vi "New Test.vi"(8 "error in (no error)":errorcluster) -> (0 "error out":errorcluster)   [LabVIEW 2020, in "MacroAssert.lvlib"]
doc: "Presents an interface to create, edit, save, and execute user-defined macros."
uses:
  MacroAssert.lvlib
  <vilib>/Utility/miscctls.llb/LVRowAndColumnUnsignedTypeDef.ctl
  bd503c13-d10c-440e-ab5e-4e60baef5deb.vi
  SubVIs/FaKI State Machine/FaKI State Machine.lvlib
  CTLs/State Data.ctl
  CTLs/Hotkey Values.ctl
  CTLs/FGV Actions.ctl
  CTLs/Hotkey Type.ctl
  CTLs/Refs.ctl
  CTLs/Step Type V3.ctl
  CTLs/Step V3.ctl
  CTLs/Macro Cluster V3.ctl
  CTLs/Macro Config V3.ctl
  fa5aba67-e91f-4216-ac5c-c17457851557.vi
  CTLs/Assertion Type.ctl
  CTLs/Report Data.ctl
  <vilib>/Utility/inputDevices.llb/closeKeyboard.vi
panel:
  in  "String":string="C:\\Users\\User\\Desktop\\test.txt"
  in  "File Path":path
  out "Status":string
  in  "Add Step 2":bool
  in  "Dbl Click":T1
  in  "Macro Steps":i32(listbox)
  out "Abort Hotkey":string caption="Abort Hotkey:"
  out "Metadata":string
  in  "Description":string
  out "Resolutions":cluster{"Width":i16, "Height":i16}[](array[cluster])
  out "n Monitors":i32
  in  "Settings":bool
  in  "Export":bool
  in  "Import":bool
  out "Macro Hotkey":string caption="Macro Hotkey:"
  in  "Delete":bool
  in  "Start/Stop":bool
  in  "N":i32 caption="Times to Repeat\n(-1 = indefinitely)" min=-1
  in  "Activation Type":enum32{"Hotkey", "Automatic"}(radio)
  out "Row":i32
  in  "Clear Steps":bool
  in  "Delete Step":bool
  in  "Insert Step":bool
  in  "Add Step":bool
  in  "Modify Step":bool
  in  "Exit":bool
  in  "Save":bool
  in  "Restore":bool
  in  "Help":bool
  in  "Macro Name":string(combo)
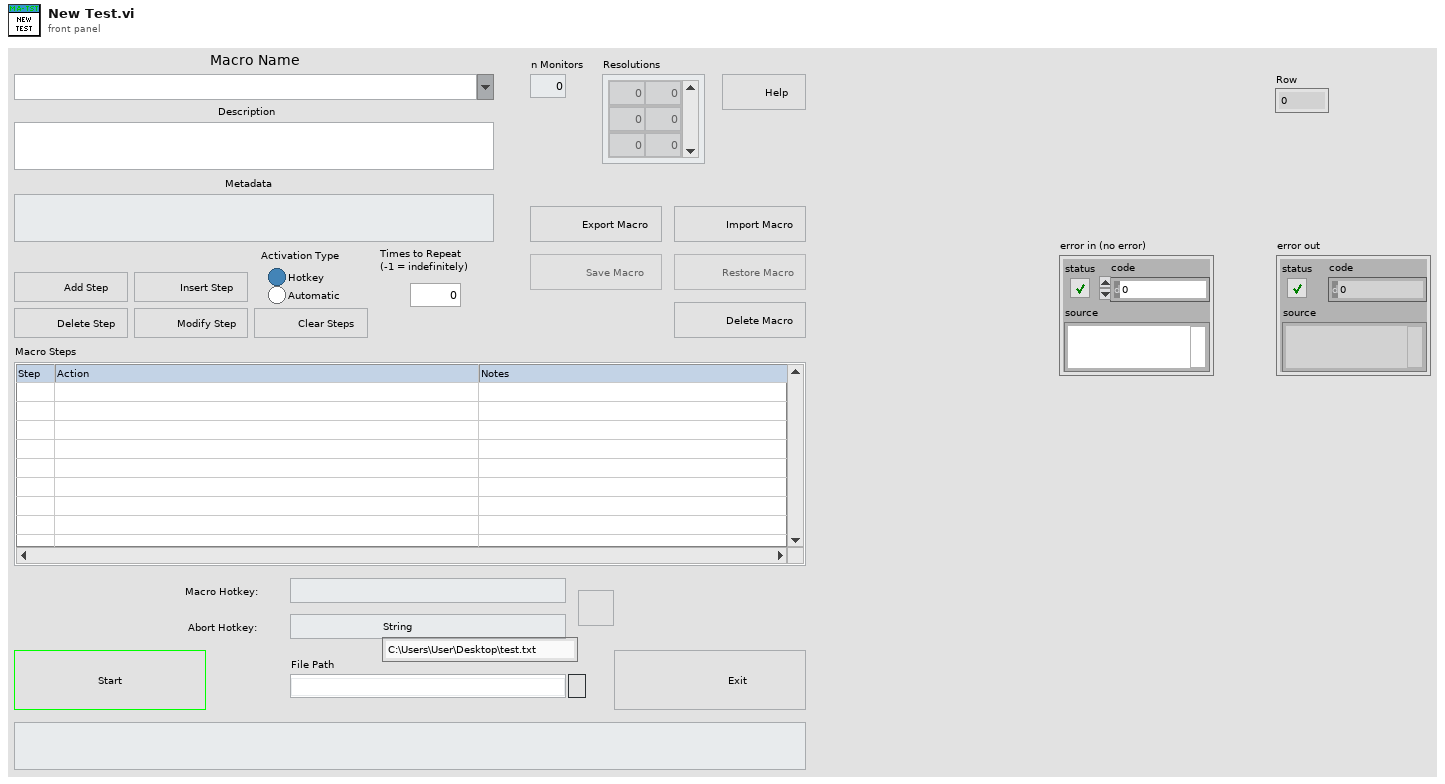
[diagram p1: front panel]
types:
  T1 = cluster{"Insert Before":bool, "Insert After":bool, "Modify Step 2":bool, "Delete Step 2":bool}
  T2 = typedef "LVPoint32TypeDef.ctl" = cluster{"Horizontal":i32, "Vertical":i32}
  T3 = enum32{"Invalid", "Standard", "Closed", "Hidden", "Minimized", "Maximized"}
  T4 = enum32{"invalid app kind", "Development System", "Run Time System", "Student Edition", "Embedded LabVIEW", "Evaluation", "Custom"}
  T5 = typedef "MacroAssert.lvlib/State Data.ctl" = cluster{"Core":cluster{"Current VI Reference":refnum<vi>, "Close Panel on Exit?":bool}, "Macro":cluster{"New":T6, "Saved":T6, "Name":string}, "Step":i32, "n":i32, "Hotkey Values":T11, "Keyboard":refnum<k1>, "Macro Active?":bool, "Macro Names":string[], "Rcount":i32, "Refs":T12, "Resolutions":cluster{"Width":i16, "Height":i16}[], "App Data Dir":path, "Start Time":timestamp, "Report Data":T13[]}
  T6 = typedef "MacroAssert.lvlib/Macro Cluster V3.ctl" = cluster{"Config":T7, "Steps":T8[]}
  T7 = typedef "MacroAssert.lvlib/Macro Config V3.ctl" = cluster{"Schema Version":string, "Activation Type":enum32{"Hotkey", "Automatic"}, "N":i32, "Description":string, "Resolutions":cluster{"Width":i16, "Height":i16}[], "Date Created":timestamp, "Date Updated":timestamp}
  T8 = typedef "MacroAssert.lvlib/Step V3.ctl" = cluster{"Type":T9, "X":i32, "Y":i32, "Delay":i32, "Key":u8, "Repeat":i32, "RClick?":bool, "App/Window Name":string, "Notes":string, "Assertion Type":T10, "Assertion Parameters":variant}
  T9 = typedef "MacroAssert.lvlib/Step Type V3.ctl" = enum16{"Mouse Move", "Mouse Click", "Key Press", "Wait", "Mouse Down", "Mouse Up", "Key Down", "Key Up", "Test Assertion", "Run Application", "Maximize Window", "Restore Window", "Minimize Window", "Close Window", "Bring Window to Front", "Send Window to Back"}
  T10 = typedef "MacroAssert.lvlib/Assertion Type.ctl" = enum16{"Control Position", "Control Visible", "Control Disabled", "Control Image"}
  T11 = typedef "MacroAssert.lvlib/Hotkey Values.ctl" = cluster{"Macro Hotkey":enum16{"0", "1", "2", "3", "4", "5", "6", "7", "8", "9", "A", "B", "C", "D", "E", "F", "G", "H", "I", "J", "K", "L", "M", "N", "O", "P", "Q", "R", "S", "T", "U", "V", "W", "X", "Y", "Z", "F1", "F2", "F3", "F4", "F5", "F6", "F7", "F8", "F9", "F10", "F11", "F12", "F13", "F14", "F15", "ADD", "BACK", "BACKSLASH", "CAPITAL", "COMMA", "DECIMAL", "DELETE", "DIVIDE", "DOWN", "END", "EQUALS", "ESCAPE", "GRAVE (`)", "HOME", "INSERT", "LBRACKET", "LCONTROL", "LEFT", "L ALT", "LSHIFT", "LWIN", "MINUS", "MULTIPLY", "NEXT", "NUMLOCK", "NUMPAD_0", "NUMPAD_1", "NUMPAD_2", "NUMPAD_3", "NUMPAD_4", "NUMPAD_5", "NUMPAD_6", "NUMPAD_7", "NUMPAD_8", "NUMPAD_9", "PAUSE", "PERIOD", "PRIOR (PG UP)", "RBRACKET", "RCONTROL", "RETURN", "RIGHT", "R ALT", "RSHIFT", "RWIN", "SCROLL", "SEMICOLON", "SLASH", "SPACE", "SUBTRACT", "TAB", "UP", "ENTER (num pad)", "' (quote)"}[], "Abort Hotkey":enum16{"0", "1", "2", "3", "4", "5", "6", "7", "8", "9", "A", "B", "C", "D", "E", "F", "G", "H", "I", "J", "K", "L", "M", "N", "O", "P", "Q", "R", "S", "T", "U", "V", "W", "X", "Y", "Z", "F1", "F2", "F3", "F4", "F5", "F6", "F7", "F8", "F9", "F10", "F11", "F12", "F13", "F14", "F15", "ADD", "BACK", "BACKSLASH", "CAPITAL", "COMMA", "DECIMAL", "DELETE", "DIVIDE", "DOWN", "END", "EQUALS", "ESCAPE", "GRAVE (`)", "HOME", "INSERT", "LBRACKET", "LCONTROL", "LEFT", "L ALT", "LSHIFT", "LWIN", "MINUS", "MULTIPLY", "NEXT", "NUMLOCK", "NUMPAD_0", "NUMPAD_1", "NUMPAD_2", "NUMPAD_3", "NUMPAD_4", "NUMPAD_5", "NUMPAD_6", "NUMPAD_7", "NUMPAD_8", "NUMPAD_9", "PAUSE", "PERIOD", "PRIOR (PG UP)", "RBRACKET", "RCONTROL", "RETURN", "RIGHT", "R ALT", "RSHIFT", "RWIN", "SCROLL", "SEMICOLON", "SLASH", "SPACE", "SUBTRACT", "TAB", "UP", "ENTER (num pad)", "' (quote)"}[]}
  T12 = typedef "MacroAssert.lvlib/Refs.ctl" = cluster{"Name":refnum<vi>, "Description":refnum<vi>, "Import":refnum<vi>, "Export":refnum<vi>, "Delete":refnum<vi>, "Restore":refnum<vi>, "Save":refnum<vi>, "Start":refnum<vi>, "Steps":refnum<vi>, "Simple Refs":refnum<vi>[]}
  T13 = typedef "MacroAssert.lvlib/Report Data.ctl" = cluster{"Step":string, "Pass?":bool, "Actual Value":variant}
  T14 = enum8{"Enabled", "Disabled", "Disabled and Grayed Out"}
  T15 = typedef "LVRowAndColumnUnsignedTypeDef.ctl" = cluster{"Row":u32, "Column":u32}
  T16 = typedef "MacroAssert.lvlib/Hotkey Type.ctl" = enum16{"Macro Hotkey", "Abort Hotkey"}
  T17 = typedef "MacroAssert.lvlib/FGV Actions.ctl" = enum16{"Read", "Write"}
  T18 = cluster{"Current VI Reference":refnum<vi>, "Close Panel on Exit?":bool}
  T19 = enum16{"0", "1", "2", "3", "4", "5", "6", "7", "8", "9", "A", "B", "C", "D", "E", "F", "G", "H", "I", "J", "K", "L", "M", "N", "O", "P", "Q", "R", "S", "T", "U", "V", "W", "X", "Y", "Z", "F1", "F2", "F3", "F4", "F5", "F6", "F7", "F8", "F9", "F10", "F11", "F12", "F13", "F14", "F15", "ADD", "BACK", "BACKSLASH", "CAPITAL", "COMMA", "DECIMAL", "DELETE", "DIVIDE", "DOWN", "END", "EQUALS", "ESCAPE", "GRAVE (`)", "HOME", "INSERT", "LBRACKET", "LCONTROL", "LEFT", "L ALT", "LSHIFT", "LWIN", "MINUS", "MULTIPLY", "NEXT", "NUMLOCK", "NUMPAD_0", "NUMPAD_1", "NUMPAD_2", "NUMPAD_3", "NUMPAD_4", "NUMPAD_5", "NUMPAD_6", "NUMPAD_7", "NUMPAD_8", "NUMPAD_9", "PAUSE", "PERIOD", "PRIOR (PG UP)", "RBRACKET", "RCONTROL", "RETURN", "RIGHT", "R ALT", "RSHIFT", "RWIN", "SCROLL", "SEMICOLON", "SLASH", "SPACE", "SUBTRACT", "TAB", "UP", "ENTER (num pad)", "' (quote)"}[]
  T20 = typedef "LVAllMonitorsDisplayTypeDef.ctl" = cluster{"Bounds":cluster{"Left":i16, "Top":i16, "Right":i16, "Bottom":i16}, "Depth":i16}[]
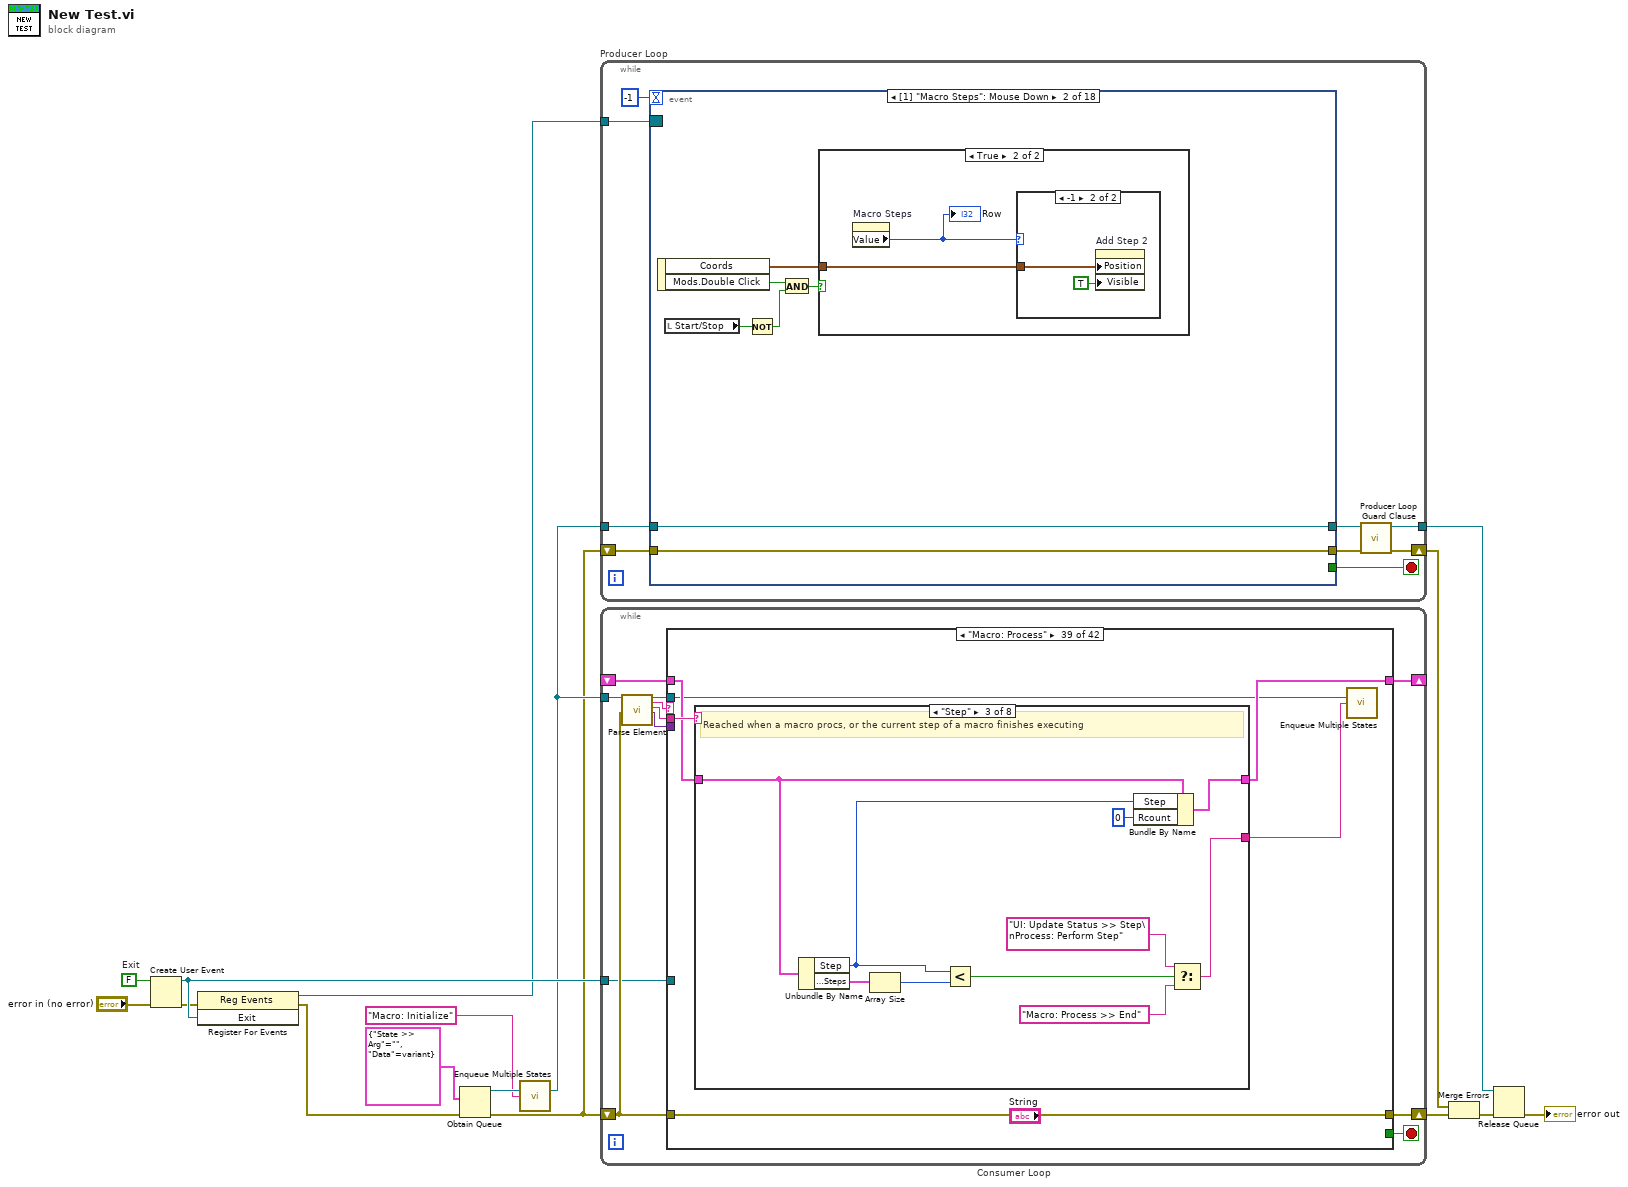
[diagram p0: block diagram]
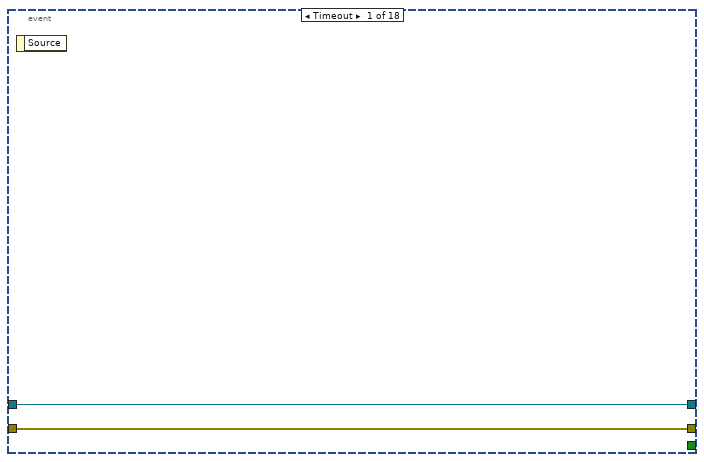
[diagram p2: hidden frame]
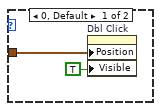
[diagram p4: hidden frame]
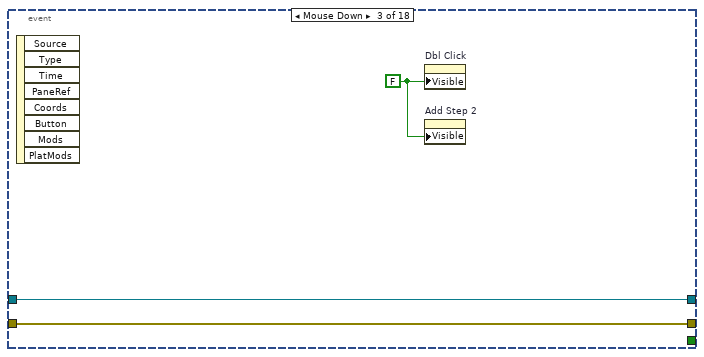
[diagram p5: hidden frame]
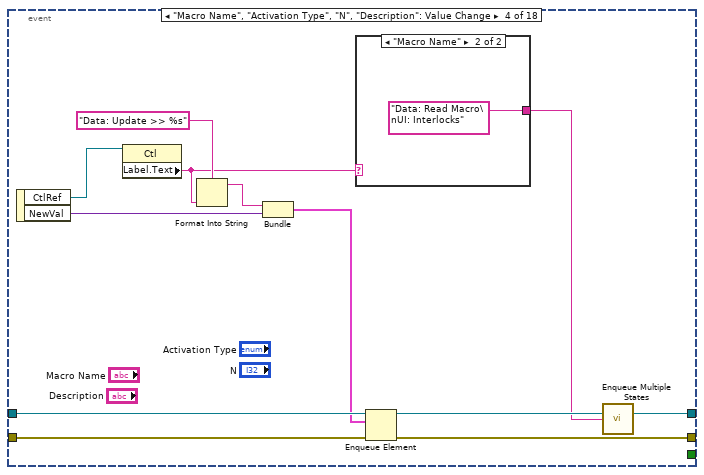
[diagram p6: hidden frame]
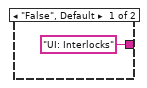
[diagram p7: hidden frame]
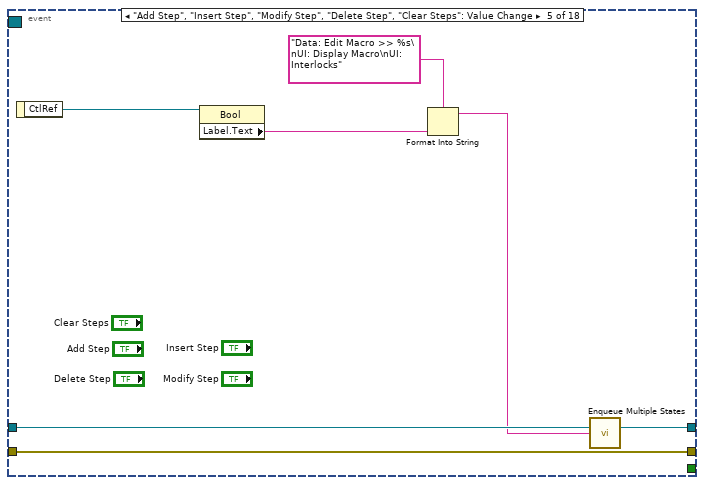
[diagram p8: hidden frame]
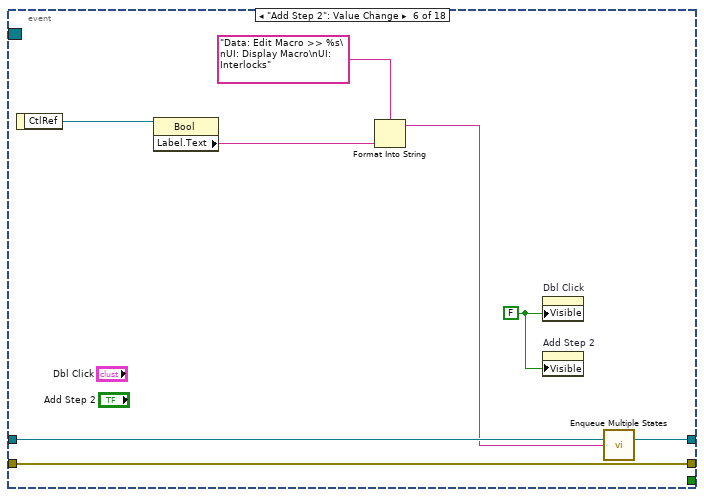
[diagram p9: hidden frame]
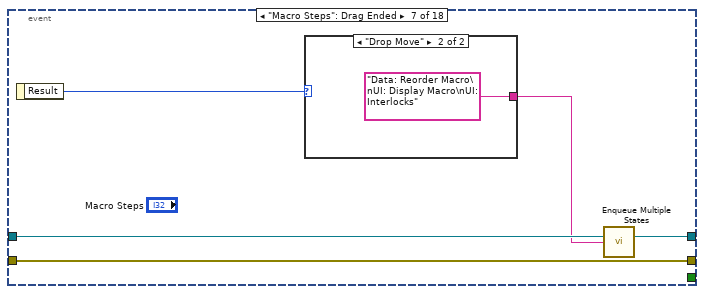
[diagram p10: hidden frame]
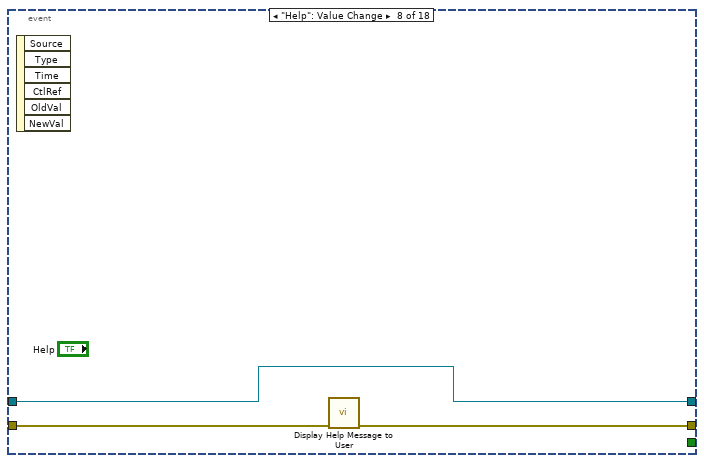
[diagram p12: hidden frame]
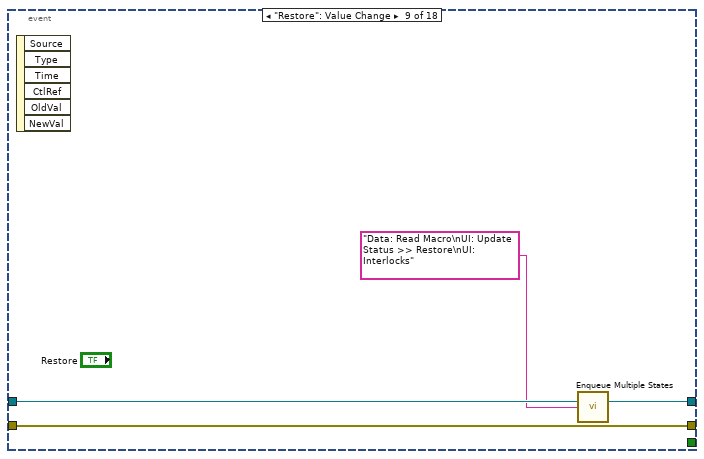
[diagram p13: hidden frame]
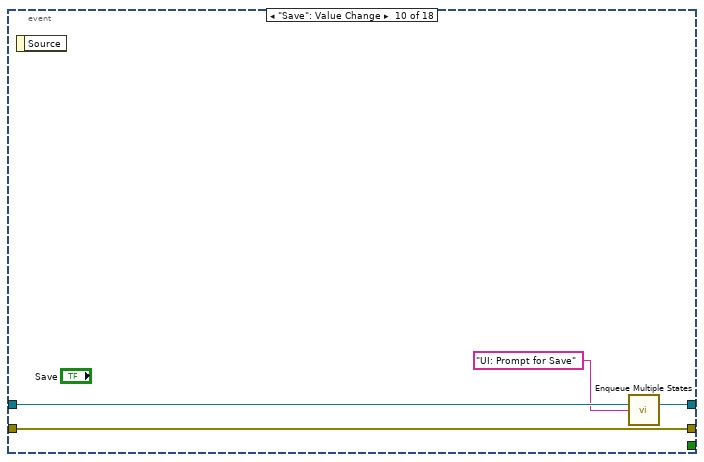
[diagram p14: hidden frame]
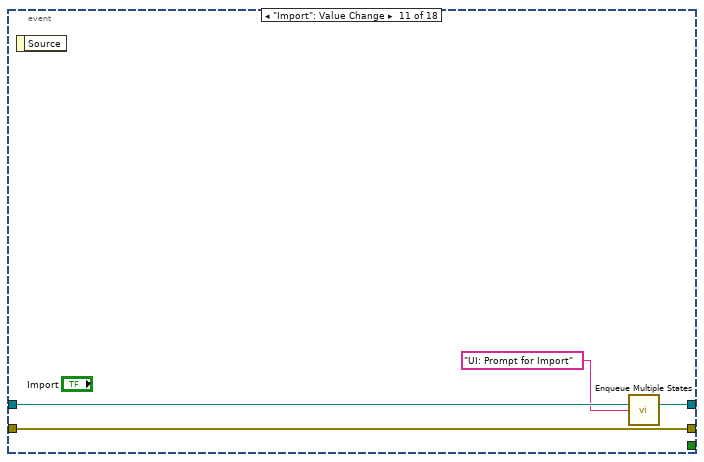
[diagram p15: hidden frame]
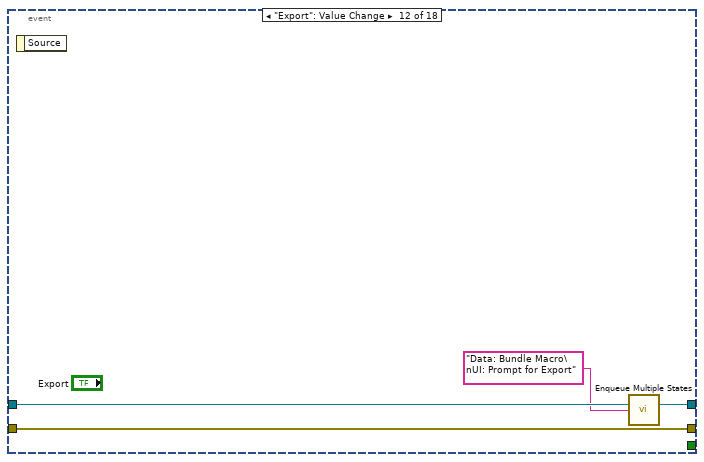
[diagram p16: hidden frame]
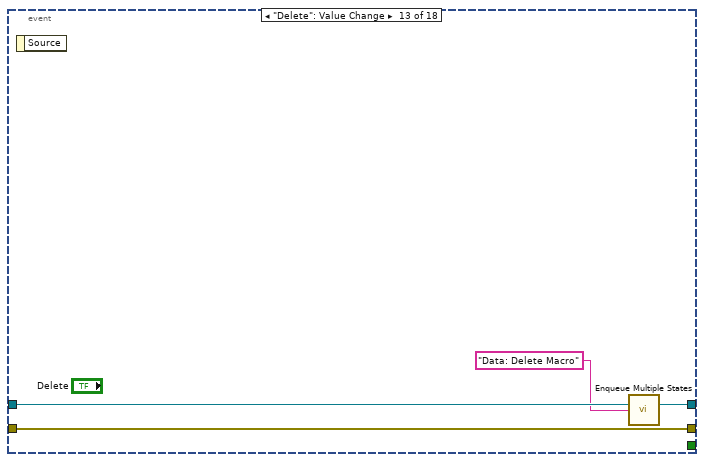
[diagram p17: hidden frame]
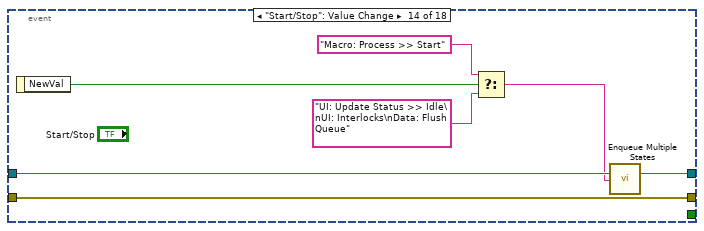
[diagram p18: hidden frame]
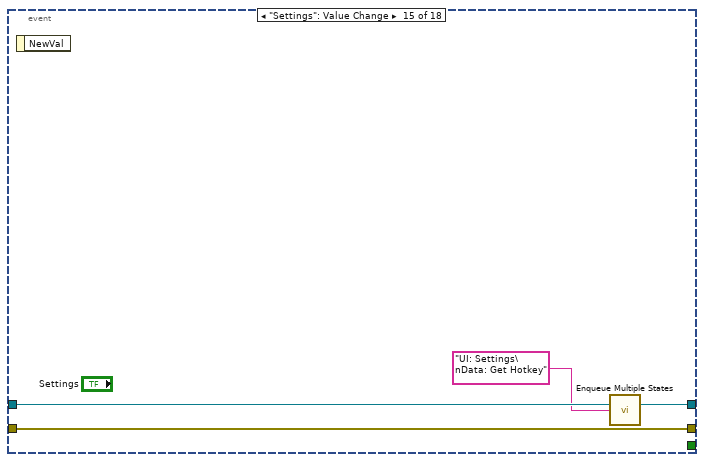
[diagram p19: hidden frame]
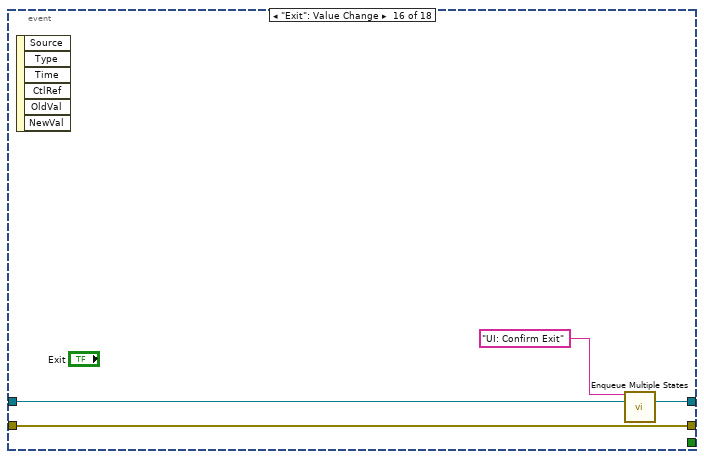
[diagram p20: hidden frame]
diagram:
  w13 = FALSE  # Exit
  n1 = Create User Event(user event datatype=w13, error in="error in (no error)") -> (user event=w16:refnum<user-event>, error out=w12:errorcluster)
  n2 = register-events(error in=w12, w16) -> (reference out=w15:refnum<event-registration>, error out=w14:errorcluster)  [unwired: 1 in]
  n3 = Obtain Queue(element data type=cluster{"State >> Arg":string, "Data":variant} {"State >> Arg"="", "Data"=variant}, error in (no error)=w14) -> (queue out=w6:refnum<queue>, error out=w3:errorcluster)  [unwired: 3 in, 1 out]
  n4 = call "Enqueue Multiple States.vi"("queue in"=w6, "State(s) at Back"="Macro: Initialize") -> ("queue out"=w7:refnum<queue>)  [unwired: 13 in]
  n5 = while "Producer Loop" {
    shift-right: [w25] -> w9
    shift-left: w3 -> [w23]
    tunnel: w15 -> [w19]
    tunnel: w7 -> [w21]
    tunnel: [w24] -> w11
    stop <- w18 stop-if-true
    n6 = event shown="[1] \"Macro Steps\": Mouse Down" {
      selector: w19 -> [_ _ _ _ _ _ _ _ _ _ _ _ _ _ _ _ _ _]
      dyn-events: _ -> [_ _ _ _ _ _ _ _ _ _ _ _ _ _ _ _ _ _]
      timeout: -1 ("Timeout") -> [_ _ _ _ _ _ _ _ _ _ _ _ _ _ _ _ _ _]
      tunnel: [w27 w34 w43 w51 w64 w72 w77 w80 w85 w89 w93 w97 w101 w108 w112 w116 w122 w127] -> w22
      tunnel: w23 -> [w27 w34 w43 w54 w64 w72 w77 w81 w85 w89 w93 w97 w101 w108 w112 w116 w122 w127]
      tunnel: w21 -> [w26 w32 w42 w48 w62 w69 w76 w79 w83 w88 w92 w96 w100 w104 w110 w114 w119 w125]
      tunnel: [w26 w32 w42 w53 w61 w68 w75 w79 w84 w87 w91 w95 w99 w105 w111 w113 w118 w124] -> w20
      tunnel: [_ _ _ _ _ _ _ _ _ _ _ _ _ _ _ _ FALSE TRUE] -> w18
      event Timeout {
        n7 = event-data() -> ()  [unwired: 1 in, 1 out]
      }
      event "Macro Steps": Mouse Down {
        n8 = event-data() -> ("Coords"=w33:T2, "Mods.Double Click"=w29:bool)  [unwired: 1 in]
        n9 = local read "Start/Stop"() -> (w31:bool)
        n10 = Not(x=w31) -> (.not. x?=w30:bool)
        n11 = And(x=w29, y=w30) -> (x .and. y?=w28:bool)
        n12 = case shown="True" w28 {
          tunnel: w33 -> [_ w36]
          frame False {
          }
          frame True {
            n13 = property on="Macro Steps" class="MCListbox (strict)"() -> ("Value"=w35:i32)  [unwired: 2 in, 2 out]
            "Row" <- w35
            n14 = case shown="-1" w35 {
              tunnel: w36 -> [w37 w39]
              frame 0, Default {
                n15 = property on="Dbl Click" class="Clust"("Position"=w37, "Visible"=TRUE) -> ()  [unwired: 2 in, 2 out]
              }
              frame -1 {
                n16 = property on="Add Step 2" class="Bool"("Position"=w39, "Visible"=TRUE) -> ()  [unwired: 2 in, 2 out]
              }
            }
          }
        }
      }
      event Mouse Down {
        w41 = FALSE ("Visible")
        n17 = event-data() -> ()  [unwired: 1 in, 8 out]
        n18 = property on="Dbl Click" class="Clust"("Visible"=w41) -> ()  [unwired: 2 in, 2 out]
        n19 = property on="Add Step 2" class="Bool"("Visible"=w41) -> ()  [unwired: 2 in, 2 out]
      }
      event "Macro Name", "Activation Type", "N", "Description": Value Change {
        n20 = event-data() -> ("CtlRef"=w50:refnum<vi>, "NewVal"=w46:variant)  [unwired: 1 in]
        n21 = property class="Ctl"(reference=w50) -> ("Label.Text"=w45:string)  [unwired: 1 in, 2 out]
        n22 = Format Into String(format string="Data: Update >> %s", w45) -> (resulting string=w47:string)  [unwired: 2 in, 1 out]
        n23 = Bundle(w47, "NewVal"=w46) -> (w44:cluster{string, "NewVal":variant})  [unwired: 1 in]
        n24 = case shown="\"Macro Name\"" w45 {
          tunnel: ["UI: Interlocks" ("string") "Data: Read Macro\nUI: Interlocks" ("string")] -> w52
          frame "False", Default {
          }
          frame "Macro Name" {
          }
        }
        n25 = Enqueue Element(queue=w48, element=w44, error in (no error)=w54) -> (queue out=w55:refnum<queue>, error out=w51:errorcluster)  [unwired: 1 in, 1 out]
        n26 = call "Enqueue Multiple States.vi"("queue in"=w55, "State(s) at Back"=w52) -> ("queue out"=w53:refnum<queue>)  [unwired: 13 in]
      }
      event "Add Step", "Insert Step", "Modify Step", "Delete Step", "Clear Steps": Value Change {
        n27 = event-data() -> ("CtlRef"=w63:refnum<vi>)  [unwired: 1 in]
        n28 = property class="Bool"(reference=w63) -> ("Label.Text"=w60:string)  [unwired: 1 in, 2 out]
        n29 = Format Into String(format string="Data: Edit Macro >> %s\nUI: Display Macro\nUI: Interlocks", w60) -> (resulting string=w58:string)  [unwired: 2 in, 1 out]
        n30 = call "Enqueue Multiple States.vi"("queue in"=w62, "State(s) at Back"=w58) -> ("queue out"=w61:refnum<queue>)  [unwired: 13 in]
      }
      event "Dbl Click.Insert Before", "Dbl Click.Insert After", "Dbl Click.Modify Step 2", "Dbl Click.Delete Step 2", "Add Step 2": Value Change {
        w70 = FALSE ("Visible")
        n31 = event-data() -> ("CtlRef"=w71:refnum<vi>)  [unwired: 1 in]
        n32 = property class="Bool"(reference=w71) -> ("Label.Text"=w66:string)  [unwired: 1 in, 2 out]
        n33 = Format Into String(format string="Data: Edit Macro >> %s\nUI: Display Macro\nUI: Interlocks", w66) -> (resulting string=w65:string)  [unwired: 2 in, 1 out]
        n34 = property on="Dbl Click" class="Clust"("Visible"=w70) -> ()  [unwired: 2 in, 2 out]
        n35 = property on="Add Step 2" class="Bool"("Visible"=w70) -> ()  [unwired: 2 in, 2 out]
        n36 = call "Enqueue Multiple States.vi"("queue in"=w69, "State(s) at Back"=w65) -> ("queue out"=w68:refnum<queue>)  [unwired: 13 in]
      }
      event "Macro Steps": Drag Ended {
        n37 = event-data() -> ("Result"=w73:enum16{"Drop Cancel", "Drop Move", "Drop Copy"})  [unwired: 1 in]
        n38 = case shown="\"Drop Move\"" w73 {
          tunnel: [_ "Data: Reorder Macro\nUI: Display Macro\nUI: Interlocks" ("State(s) at Back")] -> w74
          frame "Drop Cancel", Default {
          }
          frame "Drop Move" {
          }
        }
        n39 = call "Enqueue Multiple States.vi"("queue in"=w76, "State(s) at Back"=w74) -> ("queue out"=w75:refnum<queue>)  [unwired: 13 in]
      }
      event "Help": Value Change {
        n40 = event-data() -> ()  [unwired: 1 in, 6 out]
        n41 = call "Display Help Message to User"("error in (no error)"=w81) -> ("error out"=w80:errorcluster)  [unwired: 9 in, 1 out]
      }
      event "Restore": Value Change {
        n42 = event-data() -> ()  [unwired: 1 in, 6 out]
        n43 = call "Enqueue Multiple States.vi"("queue in"=w83, "State(s) at Back"="Data: Read Macro\nUI: Update Status >> Restore\nUI: Interlocks" ("State(s) at Back (\"\")")) -> ("queue out"=w84:refnum<queue>)  [unwired: 13 in]
      }
      event "Save": Value Change {
        n44 = event-data() -> ()  [unwired: 1 in, 1 out]
        n45 = call "Enqueue Multiple States.vi"("queue in"=w88, "State(s) at Back"="UI: Prompt for Save" ("State(s) at Back (\"\")")) -> ("queue out"=w87:refnum<queue>)  [unwired: 13 in]
      }
      event "Import": Value Change {
        n46 = event-data() -> ()  [unwired: 1 in, 1 out]
        n47 = call "Enqueue Multiple States.vi"("queue in"=w92, "State(s) at Back"="UI: Prompt for Import" ("State(s) at Back (\"\")")) -> ("queue out"=w91:refnum<queue>)  [unwired: 13 in]
      }
      event "Export": Value Change {
        n48 = event-data() -> ()  [unwired: 1 in, 1 out]
        n49 = call "Enqueue Multiple States.vi"("queue in"=w96, "State(s) at Back"="Data: Bundle Macro\nUI: Prompt for Export" ("State(s) at Back (\"\")")) -> ("queue out"=w95:refnum<queue>)  [unwired: 13 in]
      }
      event "Delete": Value Change {
        n50 = event-data() -> ()  [unwired: 1 in, 1 out]
        n51 = call "Enqueue Multiple States.vi"("queue in"=w100, "State(s) at Back"="Data: Delete Macro" ("State(s) at Back (\"\")")) -> ("queue out"=w99:refnum<queue>)  [unwired: 13 in]
      }
      event "Start/Stop": Value Change {
        n52 = event-data() -> ("NewVal"=w107:bool)  [unwired: 1 in]
        n53 = Select(t="Macro: Process >> Start", s=w107, f="UI: Update Status >> Idle\nUI: Interlocks\nData: Flush Queue") -> (s? t:f=w103:string)
        n54 = call "Enqueue Multiple States.vi"("queue in"=w104, "State(s) at Back"=w103) -> ("queue out"=w105:refnum<queue>)  [unwired: 13 in]
      }
      event "Settings": Value Change {
        n55 = event-data() -> ()  [unwired: 1 in, 1 out]
        n56 = call "Enqueue Multiple States.vi"("queue in"=w110, "State(s) at Back"="UI: Settings\nData: Get Hotkey" ("f")) -> ("queue out"=w111:refnum<queue>)  [unwired: 13 in]
      }
      event "Exit": Value Change {
        n57 = event-data() -> ()  [unwired: 1 in, 6 out]
        n58 = call "Enqueue Multiple States.vi"("State(s) at Front"="UI: Confirm Exit", "queue in"=w114) -> ("queue out"=w113:refnum<queue>)  [unwired: 13 in]
      }
      event Panel Close? {
        # "Discard the event because we'll close the front panel ourselves in Macro: Exit"
        n59 = event-data() -> ()  [unwired: 1 in, 1 out]
        n60 = call "Enqueue Multiple States.vi"("State(s) at Front"="UI: Confirm Exit", "queue in"=w119) -> ("queue out"=w118:refnum<queue>)  [unwired: 13 in]
        n61 = event-data("Discard?"=TRUE) -> ()  [unwired: 1 in, 1 out]
      }
      event User Event {
        n62 = event-data() -> ()  [unwired: 1 in, 5 out]
        n63 = call "Enqueue Multiple States.vi"("State(s) at Front"="Macro: Exit", "queue in"=w125) -> ("queue out"=w124:refnum<queue>)  [unwired: 13 in]
      }
    }
    n64 = call "Producer Loop Guard Clause.vi"("error in (no error)"=w22, "queue in"=w20) -> ("error out"=w25:errorcluster, "queue out"=w24:refnum<queue>)  [unwired: 8 in]
  }
  n65 = while "Consumer Loop" {
    shift-right: [w129] -> _
    shift-left: _ -> [w134]
    shift-right: [w136] -> w8
    shift-left: w3 -> [w137]
    tunnel: w7 -> [w138]
    tunnel: w16 -> [w128]
    stop <- w135 stop-if-true
    n66 = call "Parse Element.vi"("queue in"=w138, "error in (no error)"=w137) -> ("queue out"=w133:refnum<queue>, "State"=w132:string, "Arg"=w131:string, "Data"=w130:variant)  [unwired: 14 in]
    n67 = case shown="\"Macro: Process\"" w132 {
      selector: w132 -> [_ w141 _ _ _ _ _ _ _ _ _ _ _ _ _ _ _ _ _ _ _ _ _ _ _ _ _ _ _ _ _ _ _ _ _ _ _ _ _ _ _ _]
      tunnel: w133 -> [_ _ _ _ _ _ _ _ _ _ _ _ _ _ _ _ _ w362 w385 w398 _ _ _ _ _ _ _ _ _ w571 w586 _ w609 w621 w642 _ _ w668 w669 w741 _ w762]
      tunnel: w131 -> [_ _ _ w162 _ _ _ _ _ w215 _ _ _ w278 _ _ _ _ _ _ _ _ _ w426 w434 _ _ _ w524 _ _ _ _ _ _ _ _ _ w673 _ _ _]
      tunnel: w134 -> [w139 w143 w155 w165 w169 w170 _ w193 w205 w216 w256 w270 w273 w279 w329 w334 w350 w358 w382 w399 w407 w408 w412 w429 w436 w506 w511 w522 w525 w570 w589 w597 w608 w613 w634 w657 w663 w666 w670 w746 w748 w755]
      tunnel: [w140 w145 w159 errorcluster {"status"=FALSE, "code"=0, "source"=""} ("error out") w168 w171 w173 w194 w206 w211 w257 w268 w275 w281 w331 w341 w351 w360 w386 w400 w405 w409 w416 w427 w437 w507 w513 w517 w526 w564 w585 w595 w601 w614 w636 w651 w664 w667 w674 w747 w749 w760] -> w136
      tunnel: w137 -> [w140 w144 w159 w164 w168 w171 w179 w194 w204 w214 w257 w262 w276 w281 w331 w341 w352 w361 w387 w400 w404 w409 w416 w428 w438 w507 w514 w517 w526 w573 w590 w596 w601 w615 w637 w655 w664 w667 w674 w747 w749 w761]
      tunnel: [_ _ _ _ TRUE _ _ _ _ _ _ _ _ _ _ _ _ _ _ _ _ _ _ _ _ _ _ _ _ _ _ _ _ _ _ _ _ _ _ _ _ _] -> w135
      tunnel: w130 -> [_ _ _ w161 _ _ _ _ _ w213 _ _ _ _ _ _ _ _ _ _ _ _ _ _ _ _ _ _ _ _ _ _ _ _ _ _ _ _ _ _ _ _]
      tunnel: [w139 w143 w160 w165 w169 w170 w174 w192 w205 w212 w255 w269 w273 w280 w330 w340 w349 w359 w382 w399 w407 w408 w410 w429 w436 w506 w512 w522 w525 w570 w589 w597 w608 w612 w634 w657 w663 w666 w672 w746 w748 w754] -> w129
      tunnel: w128 -> [_ _ _ _ _ _ _ _ _ _ _ _ _ _ _ _ _ _ _ _ _ _ _ _ _ _ _ _ _ _ _ _ _ _ _ w649 _ _ _ _ _ _]
      frame "---------- Core ----------" {
        # "Do not put any code in this frame.\n(it is a separator no-op)"
      }
      frame Default {
        w148 = 42 items=["No error", "Argument error", "Memory is full", "Out of zone", "End of file", "File already open", "Generic file I/O error", "File not found", "File permission error", "Disk is full", "Duplicate path", "Too many files open", "System feature not enabled", "Resource file not found", "Cannot add resource", "Resource not found", "Image not found", "Image memory error", "Pen does not exist", "Config type invalid", "Config token not found", "Config parse error", "Config memory error", "Bad external code format", "Bad external code offset", "External code not present", "Null window", "Destroy window error", "Null menu", "Print aborted", "Bad print record", "Print driver error", "Windows error during printing", "Memory error during printing", "Print dialog error", "Generic print error", "Invalid device refnum", "Device not found", "Device parameter error", "Device unit error", "Cannot open device", "Device call aborted", "Generic error", "Cancelled by user", "Object ID too low", "Object ID too high", "Object not in heap", "Unknown heap", "Unknown object (invalid DefProc)", "Unknown object (DefProc not in table)", "Message out of range", "Invalid (null) method", "Unknown message", "Manager call not supported", "Bad address", "Network operation in progress", "Network operation timed out", "Connection is busy", "Network attribute not supported", "Network error", "Address in use", "System out of memory", "Connection aborted", "Connection refused", "Not connected", "Already connected", "Connection closed", "Initialization error (interapplication manager)", "Bad occurrence", "Wait on unbound occurrence handler", "Occurrence queue overflow", "Datalog type conflict", "Unused", "Unrecognized type (interapplication manager)", "Memory corrupt", "Failed to make temporary DLL", "Old CIN version", "Drag socket not found", "Failed to load drop-object", "Failed to register OLE object", "Failed to release OLE object", "Format specifier type mismatch", "Unknown format specifier", "Too few format specifiers", "Too many format specifiers", "Scan failed", "Newer CIN version", "Error converting to variant", "Runtime menu error", "Password tampered", "Variant attribute not found", "Incompatible variant data type", "Event data is not available", "Event Store is not present", "Occurrence is not found", "Event Queue is not created", "Event info is not available", "Refnum passed is NULL", "Error retrieving Class GUID", "Error retrieving CoClass GUID", "Error retrieving TypeLib GUID.", "Bad built application magic bytes.", "Specific driver is different from the specific driver associated with the Logical Name.", "There is no session opened to the class driver.", "Max Error", "MAX - Error with config objects", "MAX - Error loading configuration", "MAX - Group not supported"]
        # "Current State"
        # "Do not delete, rename, or modify this frame.\n(this is used to capture unhandled states and typos)"
        # "Handle mistyped state name (developer tool)"
        n68 = Format Into String(format string="Software Exception: Unhandled State \"%s\"." ("message"), error in=w144, w141) -> (resulting string=w147:string, error out=w146:errorcluster)  [unwired: 1 in]
        n69 = call <vilib>:"Error Cluster From Error Code.vi"("show call chain? (False)"=TRUE, "error in (no error)"=w146, "error message (\"\")"=w147, "error code (0)"=w148) -> ("error out"=w145:errorcluster)  [unwired: 5 in]
      }
      frame "Initialize Core Data" {
        # "Do not delete, rename, or modify this frame.\n(this is used to determine panel behavior on exit)"
        # "originally closed?"
        # "exe?"
        # "If panel starts closed or is an EXE, then close it when we exit"
        n70 = property class="VI"() -> ("FP.State"=w152:T3)  [unwired: 2 in, 2 out]
        n71 = property class="App"() -> ("App.Kind"=w158:T4)  [unwired: 2 in, 2 out]
        n72 = control-ref of="Current VI Reference"() -> (w153:refnum<vi>)
        n73 = Equal?(x=w152, y=T3."Closed" ("Front Panel Window:State")) -> (x = y?=w150:bool)
        n74 = Equal?(x=w158, y=T4."Run Time System" ("Application:Kind")) -> (x = y?=w156:bool)
        n75 = Or(x=w150, y=w156) -> (x .or. y?=w154:bool)
        n76 = Bundle By Name(cluster=w155, "Core.Current VI Reference"=w153, "Core.Close Panel on Exit?"=w154) -> (w160:T5)
      }
      frame "Error Handler" {
        # "Unhandled Error -- Display it"
        # "Handle any errors here.\nYou can also output any states to clean-up after errors occur"
        # "Clear error"
        n77 = call "Build Error Message.vi"("error in (no error)"=w164, "Data"=w161, "Arg"=w162) -> ("error out"=w163:errorcluster)  [unwired: 8 in]
        n78 = call <vilib>:"General Error Handler.vi"("error in (no error)"=w163) -> ()  [unwired: 10 in, 5 out]
      }
      frame "Exit" {
        # "Do not put any code in this frame.\n(No errors that occur here will be handled.)"
      }
      frame "---------- Data ----------" {
        # "Do not put any code in this frame.\n(It is a separator no-op. You can make a copy of this frame to create a new Data frame)"
      }
      frame "Data: Initialize" {
        w175 = T18 {"Current VI Reference"=refnum, "Close Panel on Exit?"=FALSE}  # Core
        # "Initialize the shift-register data, here."
        n79 = call <vilib>:"Intialize Keyboard.vi"("error in (no error)"=w179) -> ("error out"=w178:errorcluster, "device ID"=w176:refnum<k1>)  [unwired: 9 in]
        n80 = call "App Data Directory.vi"("error in (no error)"=w178) -> ("error out"=w173:errorcluster, "App Data Directory"=w172:path)  [unwired: 9 in]
        n81 = Bundle By Name(cluster=T5 {"Core"={"Current VI Reference"=refnum, "Close Panel on Exit?"=FALSE}, "Macro"={"New"={"Config"={"Schema Version"="", "Activation Type"=enum."Hotkey", "N"=0, "Description"="", "Resolutions"=[], "Date Created"=timestamp(0 s since 1904-01-01), "Date Updated"=timestamp(0 s since 1904-01-01)}, "Steps"=[]}, "Saved"={"Config"={"Schema Version"="", "Activation Type"=enum."Hotkey", "N"=0, "Description"="", "Resolutions"=[], "Date Created"=timestamp(0 s since 1904-01-01), "Date Updated"=timestamp(0 s since 1904-01-01)}, "Steps"=[]}, "Name"=""}, "Step"=0, "n"=0, "Hotkey Values"={"Macro Hotkey"=[], "Abort Hotkey"=[]}, "Keyboard"=refnum, "Macro Active?"=FALSE, "Macro Names"=[], "Rcount"=0, "Refs"={"Name"=refnum, "Description"=refnum, "Import"=refnum, "Export"=refnum, "Delete"=refnum, "Restore"=refnum, "Save"=refnum, "Start"=refnum, "Steps"=refnum, "Simple Refs"=[]}, "Resolutions"=[], "App Data Dir"=path "", "Start Time"=timestamp(0 s since 1904-01-01), "Report Data"=[]}, "Core"=w175, "Keyboard"=w176, "App Data Dir"=w172) -> (w174:T5)
      }
      frame "Data: Bundle Refs" {
        n82 = control-ref of="Activation Type"() -> (w197:refnum<vi>)
        n83 = control-ref of="Macro Name"() -> (w195:refnum<vi>)
        n84 = control-ref of="Add Step"() -> (w202:refnum<vi>)
        n85 = control-ref of="Delete Step"() -> (w200:refnum<vi>)
        n86 = control-ref of="Insert Step"() -> (w199:refnum<vi>)
        n87 = control-ref of="Modify Step"() -> (w201:refnum<vi>)
        n88 = control-ref of="Clear Steps"() -> (w198:refnum<vi>)
        n89 = control-ref of="Settings"() -> (w183:refnum<vi>)
        n90 = control-ref of="Help"() -> (w181:refnum<vi>)
        n91 = control-ref of="N"() -> (w196:refnum<vi>)
        n92 = control-ref of="Macro Steps"() -> (w180:refnum<vi>)
        n93 = control-ref of="Macro Name"() -> (w191:refnum<vi>)
        n94 = control-ref of="Import"() -> (w189:refnum<vi>)
        n95 = control-ref of="Export"() -> (w188:refnum<vi>)
        n96 = control-ref of="Delete"() -> (w187:refnum<vi>)
        n97 = control-ref of="Restore"() -> (w186:refnum<vi>)
        n98 = control-ref of="Save"() -> (w185:refnum<vi>)
        n99 = control-ref of="Start/Stop"() -> (w184:refnum<vi>)
        n100 = control-ref of="Description"() -> (w190:refnum<vi>)
        n101 = Build Array(w202, w200, w199, w201, w198, w197, w196, w195, w183, w181) -> (w182:refnum<vi>[])
        n102 = Bundle By Name(cluster=w193, "Refs.Name"=w191, "Refs.Description"=w190, "Refs.Import"=w189, "Refs.Export"=w188, "Refs.Delete"=w187, "Refs.Restore"=w186, "Refs.Save"=w185, "Refs.Start"=w184, "Refs.Steps"=w180, "Refs.Simple Refs"=w182) -> (w192:T5)
      }
      frame "Data: Migrate Config" {
        n103 = Unbundle By Name(w205) -> ("App Data Dir"=w203:path)
        n104 = call "Config Paths.vi"("error in (no error)"=w204) -> ("error out"=w210:errorcluster, "Process Config"=w209:path, "Global Config"=w207:path)  [unwired: 8 in]
        n105 = call "Migrate Process Config.vi"("error in (no error)"=w210, "Old Process Config"=w209, "App Data Directory"=w203) -> ("error out"=w208:errorcluster)  [unwired: 8 in]
        n106 = call "Migrate Global Config.vi"("error in (no error)"=w208, "Old Global Config"=w207, "App Data Directory"=w203) -> ("error out"=w206:errorcluster)  [unwired: 8 in]
      }
      frame "Data: Update" {
        n107 = case shown="\"Macro Name\"" w215 {
          tunnel: w216 -> [w217 w222 w230 w237 w244 w251]
          tunnel: w214 -> [w218 w226 w233 w240 w247 w254]
          tunnel: w213 -> [_ w225 w232 w239 w246 w253]
          tunnel: [w217 w221 w229 w236 w243 w250] -> w212
          tunnel: [w218 w220 w228 w235 w242 w249] -> w211
          frame "False", Default {
          }
          frame "Macro Name" {
            n108 = Variant To Data(error in=w226, type="", Variant=w225) -> (data=w223:string, error out=w220:errorcluster)
            n109 = property on="Restore" class="Bool"("DisabledEnum"=T14."Disabled and Grayed Out" ("Disabled")) -> ()  [unwired: 2 in, 2 out]
            n110 = Bundle By Name(cluster=w222, "Macro.Name"=w223) -> (w221:T5)
          }
          frame "Activation Type" {
            n111 = Variant To Data(error in=w233, type=enum32{"Hotkey", "Automatic"}."Hotkey" ("FP CTLs.Type"), Variant=w232) -> (data=w231:enum32{"Hotkey", "Automatic"}, error out=w228:errorcluster)
            n112 = Bundle By Name(cluster=w230, "Macro.New.Config.Activation Type"=w231) -> (w229:T5)
          }
          frame "N" {
            n113 = Variant To Data(error in=w240, type=0 ("FP CTLs.N"), Variant=w239) -> (data=w238:i32, error out=w235:errorcluster)
            n114 = Bundle By Name(cluster=w237, "Macro.New.Config.N"=w238) -> (w236:T5)
          }
          frame "Description" {
            n115 = Variant To Data(error in=w247, type="" ("FP CTLs.N"), Variant=w246) -> (data=w245:string, error out=w242:errorcluster)
            n116 = Bundle By Name(cluster=w244, "Macro.New.Config.Description"=w245) -> (w243:T5)
          }
          frame "Macro Active?" {
            n117 = Variant To Data(error in=w254, type=FALSE, Variant=w253) -> (data=w252:bool, error out=w249:errorcluster)
            n118 = Bundle By Name(cluster=w251, "Macro Active?"=w252) -> (w250:T5)
          }
        }
      }
      frame "Data: Increment Step" {
        n119 = in-place {
          n120 = in-place-cluster #1(w256) -> ("Step"=w259:i32)
          n121 = Increment(x=w259) -> (x+1=w258:i32)
          n122 = in-place-cluster #1("Step"=w258) -> (w255:T5)
        }
      }
      frame "Data: Get Hotkey" {
        n123 = call "App Config INI.vi"("error in (no error)"=w262) -> ("error out"=w261:errorcluster, "App Config"=w260:path)  [unwired: 9 in]
        n124 = call "Get Hotkey.vi"("error in (no error)"=w261, "File Path"=w260) -> ("error out"=w268:errorcluster, "Hotkey Values"=w266:T11)  [unwired: 8 in]
        n125 = Unbundle By Name(w266) -> ("Macro Hotkey"=w265:T19, "Abort Hotkey"=w263:T19)
        n126 = Bundle By Name(cluster=w270, "Hotkey Values"=w266) -> (w269:T5)
        n127 = call "Convert Hotkey to String.vi"("Hotkey"=w265) -> ("String"=→"Macro Hotkey":string)  [unwired: 10 in]
        n128 = call "Convert Hotkey to String.vi"("Hotkey"=w263) -> ("String"=→"Abort Hotkey":string)  [unwired: 10 in]
      }
      frame "Data: Build Report" {
        n129 = Unbundle By Name(w273) -> ("Macro.New.Steps"=w272:T8[], "Report Data"=w271:T13[])
        n130 = call "Build Report.vi"("error in (no error)"=w276, "Report Data"=w271, "Steps"=w272, "Path"="File Path") -> ("error out"=w275:errorcluster)  [unwired: 7 in]
      }
      frame "Data: Edit Macro" {
        n131 = local read "Row"() -> (w277:i32)
        n132 = in-place {
          in-place-border: w278 -> [w283]
          in-place-border: w277 -> [w282]
          n133 = in-place-cluster #2(w279) -> ("Macro.New.Steps"=w285:T8[])
          n134 = case shown="\"Clear Steps\"" w283 {
            tunnel: w285 -> [w286 w289 w292 w295 w298 w301 w305 w310 w314 w318 w320]
            tunnel: [w286 w288 w291 w294 w297 w300 w304 w309 w313 w317 w319] -> w284
            tunnel: w282 -> [_ _ _ _ _ _ w302 w307 w311 w315 _]
            frame Default {
            }
            frame "Add Step" {
              n135 = call "Alter Macro.vi"("Action"=enum16{"Add", "Insert", "Modify", "Delete"}."Add", "Steps in"=w289) -> ("Steps out"=w288:T8[])  [unwired: 9 in]
            }
            frame "Insert Step" {
              n136 = call "Alter Macro.vi"("Action"=enum16{"Add", "Insert", "Modify", "Delete"}."Insert", "Steps in"=w292) -> ("Steps out"=w291:T8[])  [unwired: 9 in]
            }
            frame "Modify Step" {
              n137 = call "Alter Macro.vi"("Action"=enum16{"Add", "Insert", "Modify", "Delete"}."Modify", "Steps in"=w295) -> ("Steps out"=w294:T8[])  [unwired: 9 in]
            }
            frame "Delete Step" {
              n138 = call "Alter Macro.vi"("Action"=enum16{"Add", "Insert", "Modify", "Delete"}."Delete", "Steps in"=w298) -> ("Steps out"=w297:T8[])  [unwired: 9 in]
            }
            frame "Add Step 2" {
              n139 = call "Alter Macro V2.vi"("Action"=enum16{"Add", "Insert", "Modify", "Delete"}."Add", "Steps in"=w301) -> ("Steps out"=w300:T8[])  [unwired: 9 in]
            }
            frame "Insert Before" {
              n140 = call "Alter Macro V2.vi"("Action"=enum16{"Add", "Insert", "Modify", "Delete"}."Insert", "Step"=w302, "Steps in"=w305) -> ("Steps out"=w304:T8[])  [unwired: 8 in]
            }
            frame "Insert After" {
              n141 = Increment(x=w307) -> (x+1=w306:i32)
              n142 = call "Alter Macro V2.vi"("Action"=enum16{"Add", "Insert", "Modify", "Delete"}."Insert", "Step"=w306, "Steps in"=w310) -> ("Steps out"=w309:T8[])  [unwired: 8 in]
            }
            frame "Modify Step 2" {
              n143 = call "Alter Macro V2.vi"("Action"=enum16{"Add", "Insert", "Modify", "Delete"}."Modify", "Step"=w311, "Steps in"=w314) -> ("Steps out"=w313:T8[])  [unwired: 8 in]
            }
            frame "Delete Step 2" {
              n144 = call "Alter Macro V2.vi"("Action"=enum16{"Add", "Insert", "Modify", "Delete"}."Delete", "Step"=w315, "Steps in"=w318) -> ("Steps out"=w317:T8[])  [unwired: 8 in]
            }
            frame "Clear Steps" {
              n145 = call "Confirm Clear"() -> ("OK"=w321:bool)  [unwired: 10 in, 1 out]
              n146 = case shown="True" w321 {
                tunnel: w320 -> [w322 _]
                tunnel: [w322 _] -> w319
                frame False {
                }
                frame True {
                  n147 = property on="Macro Steps" class="MCListbox (strict)"("TopLeft"=T15 {"Row"=0, "Column"=0} ("Index Values")) -> ()  [unwired: 2 in, 2 out]
                }
              }
            }
          }
          n148 = in-place-cluster #2("Macro.New.Steps"=w284) -> (w280:T5)
        }
      }
      frame "Data: Bundle Macro" {
        n149 = Unbundle By Name(w329) -> ("Resolutions"=w328:cluster{"Width":i16, "Height":i16}[], "Macro.New.Config.Date Created"=w326:timestamp)
        n150 = Get Date/Time In Seconds() -> (seconds since 1Jan1904=w324:timestamp)
        n151 = Not Equal To 0?(x=w326) -> (x != 0?=w327:bool)
        n152 = Select(t=w326, s=w327, f=w324) -> (s? t:f=w325:timestamp)
        n153 = Bundle By Name(cluster=w329, "Macro.New.Config.Resolutions"=w328, "Macro.New.Config.Date Created"=w325, "Macro.New.Config.Date Updated"=w324) -> (w330:T5)
      }
      frame "Data: Reorder Macro" {
        n154 = property on="Macro Steps" class="MCListbox (strict)"() -> ("ItemNames"=w339:string[][])  [unwired: 2 in, 2 out]
        n155 = Index Array(array=w339, index (col)=0 ("disabled index (col)")) -> (element=w337:string[])  [unwired: 1 in]
        n156 = Unbundle By Name(w334) -> ("Macro.New.Steps"=w333:T8[])
        n157 = Decimal String To Number(string=w337) -> (number=w336:i32[])  [unwired: 2 in, 1 out]
        n158 = Decrement(x=w336) -> (x-1=w335:i32[])
        n159 = for {
          tunnel: w335 -> [w342] mode=indexing
          tunnel: w333 -> [w344]
          tunnel: [w343] -> w332 mode=indexing
          n160 = Index Array(array=w344, index=w342) -> (element=w343:T8)
        }
        n161 = Bundle By Name(cluster=w334, "Macro.New.Steps"=w332) -> (w340:T5)
      }
      frame "Data: Save Macro" {
        n162 = Unbundle By Name(w350) -> ("Macro.New"=w348:T6, "App Data Dir"=w347:path, "Macro.Name"=w346:string)
        n163 = call "Build Path to Macro.vi"("Macro Name"=w346, "App Data Dir"=w347) -> ("Macro File Path"=w345:path)  [unwired: 9 in]
        n164 = call "Save Macro.vi"("error in (no error)"=w352, "Macro Cluster"=w348, "File Path"=w345) -> ("error out"=w351:errorcluster)  [unwired: 8 in]
        n165 = Bundle By Name(cluster=w350, "Macro.Saved"=w348) -> (w349:T5)
      }
      frame "Data: Read Macro" {
        n166 = Unbundle By Name(w358) -> ("Macro Names"=w357:string[], "Macro.Name"=w356:string, "App Data Dir"=w353:path)
        n167 = Search 1D Array(1D array=w357, element=w356) -> (index of element=w355:i32)  [unwired: 1 in]
        n168 = in-place {
          in-place-border: w361 -> [w371]
          in-place-border: [w370] -> w360
          in-place-border: w356 -> [w369]
          in-place-border: w355 -> [w368]
          in-place-border: w353 -> [w364]
          n169 = in-place-cluster #3(w358) -> ("Macro.New"=w367:T6)  [unwired: 1 out]
          n170 = case shown="0, Default" w368 {
            tunnel: w371 -> [w377 w380]
            tunnel: [w376 w380] -> w370
            tunnel: w369 -> [w373 _]
            tunnel: w367 -> [_ w379]
            tunnel: [w375 _] -> w366
            tunnel: [w375 w378] -> w365
            tunnel: w364 -> [w374 _]
            frame 0, Default {
              n171 = call "Build Path to Macro.vi"("Macro Name"=w373, "App Data Dir"=w374) -> ("Macro File Path"=w372:path)  [unwired: 9 in]
              n172 = call "Read Macro.vi"("error in (no error)"=w377, "File Path"=w372) -> ("error out"=w376:errorcluster, "Macro"=w375:T6)  [unwired: 8 in]
            }
            frame -1 {
              n173 = call "Clear Macro Data.vi"("Macro"=w379) -> ("Macro out"=w378:T6)  [unwired: 10 in]
            }
          }
          n174 = in-place-cluster #3("Macro.New"=w365, "Macro.Saved"=w366) -> (w359:T5)
        }
        n175 = property on="Macro Steps" class="MCListbox (strict)"("TopLeft"=T15 {"Row"=0, "Column"=0} ("Index Values")) -> ()  [unwired: 2 in, 2 out]
        n176 = call "Enqueue Multiple States.vi"("queue in"=w362, "State(s) at Back"="UI: Display Macro" ("State(s) at Back (\"\")")) -> ()  [unwired: 13 in, 1 out]
      }
      frame "Data: Delete Macro" {
        n177 = Unbundle By Name(w382) -> ("Macro.Name"=w383:string, "App Data Dir"=w381:path)
        n178 = call "Perm Delete?"("error in (no error)"=w387) -> ("error out"=w388:errorcluster, "Delete"=w389:bool)  [unwired: 9 in]
        n179 = case shown="True" w389 {
          tunnel: w388 -> [w390 w392]
          tunnel: [w390 w396] -> w386
          tunnel: [_ "UI: Update Status >> Delete\nUI: Populate Macros" ("State(s) at Back (\"\")")] -> w384
          tunnel: w383 -> [_ w394]
          tunnel: w381 -> [_ w393]
          frame False {
          }
          frame True {
            n180 = call "Delete Macro.vi"("Macro Name"=w394, "error in (no error)"=w392, "App Data Directory"=w393) -> ("error out"=w397:errorcluster)  [unwired: 8 in]
            n181 = property on="Macro Name" class="CmbBox"(error in=w397, "Val(Sgnl)"="") -> (error out=w396:errorcluster)  [unwired: 1 in, 1 out]
          }
        }
        n182 = call "Enqueue Multiple States.vi"("queue in"=w385, "State(s) at Back"=w384) -> ()  [unwired: 13 in, 1 out]
      }
      frame "Data: Flush Queue" {
        n183 = Flush Queue(queue=w398) -> ()  [unwired: 1 in, 3 out]
      }
      frame "Data: Cleanup" {
        # "Cleanup any data and references, here.\n(this is called automatically, by the Macro: Exit)"
        n184 = Unbundle By Name(w407) -> ("Core.Current VI Reference"=w406:refnum<vi>, "Keyboard"=w401:refnum<k1>)
        n185 = Close Reference(reference=w406, error in (no error)=w404) -> (error out=w402:errorcluster)
        n186 = call-poly <vilib>:"Close Input Device.vi"("error in (no error)"=w402, "device ID"=w401) -> ("error out"=w403:errorcluster)  [unwired: 8 in]
        n187 = invoke class="VI" method="Default Vals.Reinit All"(error in=w403) -> (error out=w405:errorcluster)  [unwired: 2 in, 2 out]
      }
      frame "---------- UI ----------" {
        # "Do not put any code in this frame.\n(It is a separator no-op. You can make a copy of this frame to create a new UI frame)"
      }
      frame "UI: Initialize" {
        w417 = T14."Disabled and Grayed Out" ("Disabled")
        # "Initialize the User Interface, here.\n(this is called automatically, by the Macro: Init)"
        n188 = property class="App"() -> ("Disp.AllMonitors"=w413:T20)  [unwired: 2 in, 2 out]
        n189 = for {
          tunnel: w413 -> [w425] mode=indexing
          tunnel: [w424] -> w411 mode=indexing
          n190 = Unbundle By Name(w425) -> ("Bounds.Right"=w423:i16, "Bounds.Left"=w421:i16, "Bounds.Bottom"=w422:i16, "Bounds.Top"=w420:i16)
          n191 = Subtract(x=w423, y=w421) -> (x-y=w418:i16)
          n192 = Subtract(x=w422, y=w420) -> (x-y=w419:i16)
          n193 = Bundle(w418, w419) -> (w424:cluster{i16, i16})  [unwired: 1 in]
        }
        "Resolutions" <- w411
        n194 = Array Size(array=w413) -> (size(s)=→"n Monitors":i32)
        n195 = property on="Start/Stop" class="Bool (strict)"("DisabledEnum"=w417) -> ()  [unwired: 2 in, 2 out]
        n196 = property on="Restore" class="Bool"("DisabledEnum"=w417) -> ()  [unwired: 2 in, 2 out]
        n197 = property on="Save" class="Bool"("DisabledEnum"=w417) -> ()  [unwired: 2 in, 2 out]
        n198 = property on="Start/Stop" class="Bool (strict)"("Colors [4]"=cluster{u32, u32}[] [{65280, 65280}, {16711680, 16711680}, {4424887, 6618880}, {4424887, 16711680}, {4424887, 12648384}, {4424887, 16761024}]) -> ()  [unwired: 2 in, 2 out]
        n199 = Bundle By Name(cluster=w412, "Resolutions"=w411) -> (w410:T5)
      }
      frame "UI: Cursor Set" {
        # "Argument"
        # "Set and Unset Cursor Busy.\n(Usage: \"UI: Cursor Set >> Busy|Idle\")"
        n200 = case shown="\"Idle\", Default" w426 {
          tunnel: w428 -> [w431 w433]
          tunnel: [w430 w432] -> w427
          frame "Idle", Default {
            n201 = call <vilib>:"Unset Busy.vi"("error in (no error)"=w431) -> ("error out"=w430:errorcluster)  [unwired: 10 in]
          }
          frame "Busy" {
            n202 = call <vilib>:"Set Busy.vi"("error in (no error)"=w433) -> ("error out"=w432:errorcluster)  [unwired: 9 in, 1 out]
          }
        }
      }
      frame "UI: Front Panel State" {
        # "Argument"
        # "Set Front Panel Open or Closed\n(Usage: \"UI: Front Panel State >> Open|Close\")"
        n203 = Unbundle By Name(w436) -> ("Core.Current VI Reference"=w435:refnum<vi>)
        n204 = case shown="\"Open\", \"Standard\", Default" w434 {
          tunnel: w438 -> [w444 w459 w470 w483 w496]
          tunnel: [w446 w460 w472 w485 w498] -> w437
          tunnel: w435 -> [w445 w457 w471 w484 w497]
          frame "Open", "Standard", Default {
            w439 = T3."Standard" ("State")
            n205 = property class="VI"(reference=w445, error in=w444) -> (reference out=w442:refnum<vi>, error out=w443:errorcluster, "FP.State"=w441:T3)
            n206 = Not Equal?(x=w441, y=w439) -> (x != y?=w440:bool)
            n207 = case shown="True" w440 {
              tunnel: [w450 w452] -> w446
              tunnel: w443 -> [w449 w452]
              tunnel: w442 -> [w448 _]
              tunnel: w439 -> [w447 _]
              frame True {
                n208 = invoke class="VI" method="FP.Open"(reference=w448, error in=w449, "Activate"=TRUE, "State"=w447) -> (error out=w450:errorcluster)  [unwired: 1 in, 4 out]
              }
              frame False {
              }
            }
          }
          frame "Close", "Closed" {
            n209 = property class="VI"(reference=w457, error in=w459) -> (reference out=w456:refnum<vi>, error out=w458:errorcluster, "FP.State"=w454:T3)
            n210 = Not Equal?(x=w454, y=T3."Closed" ("Front Panel Window:State")) -> (x != y?=w453:bool)
            n211 = case shown="True" w453 {
              tunnel: [w461 w464] -> w460
              tunnel: w458 -> [w461 w463]
              tunnel: w456 -> [_ w462]
              frame False {
              }
              frame True {
                n212 = invoke class="VI" method="FP.Close"(reference=w462, error in=w463) -> (error out=w464:errorcluster)  [unwired: 1 in, 2 out]
              }
            }
          }
          frame "Hidden", "Hide" {
            w465 = T3."Hidden" ("State")
            n213 = property class="VI"(reference=w471, error in=w470) -> (reference out=w468:refnum<vi>, error out=w469:errorcluster, "FP.State"=w467:T3)
            n214 = Not Equal?(x=w467, y=w465) -> (x != y?=w466:bool)
            n215 = case shown="True" w466 {
              tunnel: [w476 w477] -> w472
              tunnel: w469 -> [w475 w477]
              tunnel: w468 -> [w474 _]
              tunnel: w465 -> [w473 _]
              frame True {
                n216 = invoke class="VI" method="FP.Open"(reference=w474, error in=w475, "State"=w473) -> (error out=w476:errorcluster)  [unwired: 2 in, 4 out]
              }
              frame False {
              }
            }
          }
          frame "Minimize", "Minimized" {
            w478 = T3."Minimized" ("State")
            n217 = property class="VI"(reference=w484, error in=w483) -> (reference out=w481:refnum<vi>, error out=w482:errorcluster, "FP.State"=w480:T3)
            n218 = Not Equal?(x=w480, y=w478) -> (x != y?=w479:bool)
            n219 = case shown="True" w479 {
              tunnel: [w489 w490] -> w485
              tunnel: w482 -> [w488 w490]
              tunnel: w481 -> [w487 _]
              tunnel: w478 -> [w486 _]
              frame True {
                n220 = invoke class="VI" method="FP.Open"(reference=w487, error in=w488, "State"=w486) -> (error out=w489:errorcluster)  [unwired: 2 in, 4 out]
              }
              frame False {
              }
            }
          }
          frame "Maximize", "Maximized" {
            w491 = T3."Maximized" ("State")
            n221 = property class="VI"(reference=w497, error in=w496) -> (reference out=w494:refnum<vi>, error out=w495:errorcluster, "FP.State"=w493:T3)
            n222 = Not Equal?(x=w493, y=w491) -> (x != y?=w492:bool)
            n223 = case shown="True" w492 {
              tunnel: [w502 w503] -> w498
              tunnel: w495 -> [w501 w503]
              tunnel: w494 -> [w500 _]
              tunnel: w491 -> [w499 _]
              frame True {
                n224 = invoke class="VI" method="FP.Open"(reference=w500, error in=w501, "State"=w499) -> (error out=w502:errorcluster)  [unwired: 2 in, 4 out]
              }
              frame False {
              }
            }
          }
        }
      }
      frame "UI: Interlocks" {
        n225 = Unbundle By Name(w506) -> ("Refs"=w505:T12, "Macro"=w504:cluster{"New":T6, "Saved":T6, "Name":string})
        n226 = call "UI Interlocks.vi"("Macro"=w504, "Refs"=w505) -> ()  [unwired: 10 in]
      }
      frame "UI: Populate Macros" {
        n227 = Unbundle By Name(w511) -> ("App Data Dir"=w509:path)
        n228 = call "Read Macro Names.vi"("error in (no error)"=w514, "App Data Directory"=w509) -> ("error out"=w513:errorcluster, "Macro Names"=w510:string[])  [unwired: 8 in]
        n229 = Sort 1D Array(array=w510) -> (sorted array=w508:string[])
        n230 = Bundle By Name(cluster=w511, "Macro Names"=w508) -> (w512:T5)
        n231 = property on="Macro Name" class="CmbBox"("Strings[]"=w508) -> ()  [unwired: 2 in, 2 out]
      }
      frame "UI: Display Macro" {
        n232 = Unbundle By Name(w522) -> ("Macro.New"=w521:T6, "Macro.New.Config.Description"=w520:string, "Macro.New.Config.Activation Type"=w519:enum32{"Hotkey", "Automatic"}, "Macro.New.Config.N"=w518:i32)
        n233 = call "Display Data to Table.vi"("Macro"=w521) -> ("Metadata"=→"Metadata":string, "Macro Steps"=w515:string[][])  [unwired: 9 in]
        n234 = local write "Description"(w520) -> ()
        n235 = local write "Activation Type"(w519) -> ()
        n236 = local write "N"(w518) -> ()
        n237 = property on="Macro Steps" class="MCListbox (strict)"("ItemNames"=w515) -> ()  [unwired: 2 in, 2 out]
      }
      frame "UI: Update Status" {
        n238 = case shown="\"Abort Listen\"" w524 {
          tunnel: w525 -> [_ _ w535 w541 w547 w553 w559 _ _ _]
          tunnel: ["Idle" "Listening for hotkey press" w529 w536 w542 w548 w554 "Macro saved" ("Status") "Macro deleted" ("Status") "Macro restored to last save" ("Status")] -> w523
          frame "Idle", Default {
          }
          frame "Listen" {
          }
          frame "Step" {
            n239 = Unbundle By Name(w535) -> ("Macro.New"=w534:T6, "Step"=w533:i32, "n"=w532:i32, "Rcount"=w531:i32, "Start Time"=w530:timestamp)
            n240 = call "Build Status Message.vi"("Start Time"=w530, "Step Repeat"=w531, "Macro Repeat"=w532, "Step"=w533, "Macro"=w534) -> ("Status"=w529:string)  [unwired: 6 in]
          }
          frame "Complete Idle" {
            n241 = Unbundle By Name(w541) -> ("Start Time"=w539:timestamp)
            n242 = Get Date/Time In Seconds() -> (seconds since 1Jan1904=w538:timestamp)
            n243 = Subtract(x=w538, y=w539) -> (x-y=w537:dbl)
            n244 = Format Into String(format string="Macro completed in %.3t s.\nIdle", w537) -> (resulting string=w536:string)  [unwired: 2 in, 1 out]
          }
          frame "Complete Listen" {
            n245 = Unbundle By Name(w547) -> ("Start Time"=w545:timestamp)
            n246 = Get Date/Time In Seconds() -> (seconds since 1Jan1904=w544:timestamp)
            n247 = Subtract(x=w544, y=w545) -> (x-y=w543:dbl)
            n248 = Format Into String(format string="Macro completed in %.3t s.\nListening for hotkey press", w543) -> (resulting string=w542:string)  [unwired: 2 in, 1 out]
          }
          frame "Abort Idle" {
            n249 = Unbundle By Name(w553) -> ("Start Time"=w551:timestamp)
            n250 = Get Date/Time In Seconds() -> (seconds since 1Jan1904=w550:timestamp)
            n251 = Subtract(x=w550, y=w551) -> (x-y=w549:dbl)
            n252 = Format Into String(format string="Macro aborted after %.3t s.\nIdle", w549) -> (resulting string=w548:string)  [unwired: 2 in, 1 out]
          }
          frame "Abort Listen" {
            n253 = Unbundle By Name(w559) -> ("Start Time"=w557:timestamp)
            n254 = Get Date/Time In Seconds() -> (seconds since 1Jan1904=w556:timestamp)
            n255 = Subtract(x=w556, y=w557) -> (x-y=w555:dbl)
            n256 = Format Into String(format string="Macro aborted after %.3t s.\nListening for hotkey press", w555) -> (resulting string=w554:string)  [unwired: 2 in, 1 out]
          }
          frame "Save" {
          }
          frame "Delete" {
          }
          frame "Restore" {
          }
        }
        "Status" <- w523
      }
      frame "UI: Wait" {
        n257 = Unbundle By Name(w570) -> ("Keyboard"=w568:refnum<k1>, "Hotkey Values"=w567:T11)
        n258 = call "Check for Hotkey Press.vi"("Hotkey Type"=Hotkey_Type."Abort Hotkey", "error in (no error)"=w573, "Hotkeys"=w567, "Keyboard"=w568) -> ("error out"=w569:errorcluster, "Pressed?"=w565:bool)  [unwired: 5 in, 1 out]
        n259 = call "Timer FGV.vi"("Mode"=FGV_Actions."Read", "error in (no error)"=w569) -> ("error out"=w576:errorcluster, "Expired?"=w574:bool)  [unwired: 7 in, 1 out]
        n260 = case "Abort pressed?" shown="False" w565 {
          tunnel: w574 -> [w580 _]
          tunnel: [w577 "Macro: Process >> Abort" ("t")] -> w572
          frame False {
            n261 = Select(t="Macro: Process >> Count", s=w580, f="UI: Wait") -> (s? t:f=w577:string)
          }
          frame True {
          }
        }
        n262 = call "Stall Data Flow.vim"("value in"=w576, "milliseconds to wait"=u32 1) -> ("value out"=w564:errorcluster)  [unwired: 1 out]
        n263 = call "Enqueue Multiple States.vi"("queue in"=w571, "State(s) at Back"=w572) -> ()  [unwired: 13 in, 1 out]
      }
      frame "UI: Listen" {
        n264 = Unbundle By Name(w589) -> ("Keyboard"=w594:refnum<k1>, "Hotkey Values"=w584:T11)
        n265 = call "Stall Data Flow.vim"("value in"=w594, "milliseconds to wait"=u32 1) -> ("value out"=w592:refnum<k1>)  [unwired: 1 out]
        n266 = call "Check for Hotkey Press.vi"("Hotkey Type"=Hotkey_Type."Macro Hotkey", "error in (no error)"=w590, "Hotkeys"=w584, "Keyboard"=w592) -> ("error out"=w585:errorcluster, "Pressed?"=w582:bool)  [unwired: 5 in, 1 out]
        n267 = Select(t="Macro: Process >> Proc", s=w582, f="UI: Listen" ("string")) -> (s? t:f=w588:string)
        n268 = call "Enqueue Multiple States.vi"("queue in"=w586, "State(s) at Back"=w588) -> ()  [unwired: 13 in, 1 out]
      }
      frame "UI: Settings" {
        n269 = call "Change Settings.vi"("error in (no error)"=w596) -> ("error out"=w595:errorcluster)  [unwired: 10 in]
      }
      frame "UI: Prompt for Save" {
        n270 = Unbundle By Name(w608) -> ("Macro Names"=w600:string[], "Macro.Name"=w599:string)
        n271 = Search 1D Array(1D array=w600, element=w599) -> (index of element=w598:i32)  [unwired: 1 in]
        n272 = Greater Or Equal To 0?(x=w598) -> (x >= 0?=w604:bool)
        n273 = call "Overwrite?"("Enable"=w604) -> ("OK"=w603:bool)  [unwired: 9 in, 1 out]
        n274 = Implies(1:w603, 2:w604) -> (0:w602:bool)
        n275 = Select(t="Data: Bundle Macro\nData: Save Macro\nUI: Populate Macros\nUI: Update Status >> Save\nUI: Interlocks", s=w602, f="") -> (s? t:f=w605:string)
        n276 = call "Enqueue Multiple States.vi"("queue in"=w609, "State(s) at Back"=w605) -> ()  [unwired: 13 in, 1 out]
      }
      frame "UI: Prompt for Import" {
        n277 = call "File Dialog"("prompt"="Select a Macro to Import", "pattern (all files)"="*.ini", "pattern label"="Configuration Files") -> ("selected path"=w616:path, "cancelled"=w610:bool, "error out"=w622:errorcluster)  [unwired: 9 in, 1 out]
        n278 = case shown="False" w610 {
          tunnel: w616 -> [w626 _]
          tunnel: w615 -> [w625 w627]
          tunnel: [w624 w627] -> w614
          tunnel: [w623 _] -> w611
          frame False {
            n279 = call "Read Macro.vi"("error in (no error)"=w625, "File Path"=w626) -> ("error out"=w624:errorcluster, "Macro"=w623:T6)  [unwired: 8 in]
          }
          frame True {
          }
        }
        n280 = call <vilib>:"Clear Errors.vi"("error in (no error)"=w622) -> ()  [unwired: 5 in, 2 out]
        n281 = in-place {
          in-place-border: w611 -> [w630]
          in-place-border: w610 -> [w631]
          n282 = in-place-cluster #4(w613) -> ("Macro.New"=w629:T6)
          n283 = Select(t=w629, s=w631, f=w630) -> (s? t:f=w628:T6)
          n284 = in-place-cluster #4("Macro.New"=w628) -> (w612:T5)
        }
        n285 = call "Enqueue Multiple States.vi"("queue in"=w621, "State(s) at Back"="UI: Display Macro\nUI: Interlocks") -> ()  [unwired: 13 in, 1 out]
      }
      frame "UI: Prompt for Export" {
        n286 = Unbundle By Name(w634) -> ("Macro.New"=w632:T6, "Macro.Name"=w633:string)
        n287 = call "File Dialog2"("prompt"="Save As", "default name"=w633, "pattern (all files)"="*.ini", "pattern label"="Configuration Files") -> ("selected path"=w638:path, "cancelled"=w635:bool, "error out"=w643:errorcluster)  [unwired: 8 in, 1 out]
        n288 = case shown="False" w635 {
          tunnel: w638 -> [w647 _]
          tunnel: w637 -> [w646 w648]
          tunnel: [w645 w648] -> w636
          tunnel: w632 -> [w644 _]
          frame False {
            n289 = call "Save Macro.vi"("error in (no error)"=w646, "Macro Cluster"=w644, "File Path"=w647) -> ("error out"=w645:errorcluster)  [unwired: 8 in]
          }
          frame True {
          }
        }
        n290 = call <vilib>:"Clear Errors.vi"("error in (no error)"=w643) -> ()  [unwired: 5 in, 2 out]
        n291 = call "Enqueue Multiple States.vi"("queue in"=w642) -> ()  [unwired: 14 in, 1 out]
      }
      frame "UI: Confirm Exit" {
        n292 = Unbundle By Name(w657) -> ("Macro.New"=w653:T6, "Macro.Saved"=w654:T6)
        n293 = Not Equal?(x=w653, y=w654) -> (x != y?=w652:bool)
        n294 = call "Exit anyway?"("Enable"=w652) -> ("Exit"=w656:bool)  [unwired: 9 in, 1 out]
        n295 = Implies(1:w656, 2:w652) -> (0:w650:bool)
        n296 = case shown="True" w650 {
          tunnel: w655 -> [w658 w662]
          tunnel: [w658 w661] -> w651
          tunnel: w649 -> [_ w660]
          frame False {
          }
          frame True {
            n297 = Generate User Event(user event=w660, event data cluster=TRUE ("event data"), error in=w662) -> (error out=w661:errorcluster)  [unwired: 1 in, 1 out]
          }
        }
      }
      frame "---------- Macro ----------" {
        # "Do not put any code in this frame.\n(It is a separator no-op. You can make a copy of this frame to create a new Macro frame)"
      }
      frame "Macro: Initialize" {
        w665 = "Data: Initialize\nData: Bundle Refs\nInitialize Core Data\nUI: Initialize\nData: Get Hotkey\nUI: Populate Macros\nUI: Interlocks\nUI: Front Panel State >> Open\nData: Migrate Config\nUI: Update Status >> Idle"  # Data: Initialize Data: Bundle Refs Initialize Core Data UI: Initialize Data: Get Hotkey UI: Populate Macros UI: Interlocks UI: Front Panel State >> Open Data: Migrate Config UI: Update Status >> Idle
        # "Initialization Macro\n(This is called once, when the VI starts)"
        n298 = call "Enqueue Multiple States.vi"("State(s) at Front"=w665, "queue in"=w668) -> ()  [unwired: 13 in, 1 out]
      }
      frame "Macro: Process" {
        n299 = case shown="\"Step\"" w673 {
          tunnel: w670 -> [w676 w684 w692 w707 w719 w725 w727 w733]
          tunnel: [w676 w687 w691 w705 w717 w724 w727 w733] -> w672
          tunnel: [w675 "UI: Interlocks\nMacro: Process >> Step" w689 w703 w715 "UI: Update Status >> Step\nProcess: Perform Step" w728 w734] -> w671
          frame "Start", Default {
            # "Reached when Start button is pressed"
            n300 = Unbundle By Name(w676) -> ("Macro.New.Config.Activation Type"=w677:enum32{"Hotkey", "Automatic"})
            n301 = Equal?(x=w677, y=enum32{"Hotkey", "Automatic"}."Hotkey") -> (x = y?=w681:bool)
            n302 = Select(t="UI: Interlocks\nUI: Update Status >> Listen\nUI: Listen", s=w681, f="Macro: Proc") -> (s? t:f=w675:string)
          }
          frame "Proc" {
            w686 = 0 ("Step")
            # "Reached when Macro hotkey is activated or right after Start button for Automatic activation type"
            n303 = Get Date/Time In Seconds() -> (seconds since 1Jan1904=w685:timestamp)
            n304 = Bundle By Name(cluster=w684, "Step"=w686, "n"=w686, "Rcount"=w686, "Start Time"=w685, "Report Data"=T13[] []) -> (w687:T5)
          }
          frame "Step" {
            # "Reached when a macro procs, or the current step of a macro finishes executing"
            n305 = Unbundle By Name(w692) -> ("Step"=w697:i32, "Macro.New.Steps"=w695:T8[])
            n306 = Array Size(array=w695) -> (size(s)=w696:i32)
            n307 = Less?(x=w697, y=w696) -> (x < y?=w694:bool)
            n308 = Bundle By Name(cluster=w692, "Step"=w697, "Rcount"=0) -> (w691:T5)
            n309 = Select(t="UI: Update Status >> Step\nProcess: Perform Step", s=w694, f="Macro: Process >> End") -> (s? t:f=w689:string)
          }
          frame "Count" {
            # "Reached when one count of the current step of a macro finishes executing"
            n310 = Unbundle By Name(w707) -> ("Rcount"=w698:i32, "Macro.New.Steps"=w702:T8[], "Step"=w701:i32)
            n311 = Index Array(array=w702, index=w701) -> (element=w700:T8)
            n312 = Unbundle By Name(w700) -> ("Repeat"=w699:i32)
            n313 = Increment(x=w698) -> (x+1=w706:i32)
            n314 = Greater Or Equal?(x=w698, y=w699) -> (x >= y?=w709:bool)
            n315 = Bundle By Name(cluster=w707, "Rcount"=w706) -> (w705:T5)
            n316 = Select(t="Data: Increment Step\nMacro: Process >> Step", s=w709, f="UI: Update Status >> Step\nProcess: Perform Step") -> (s? t:f=w703:string)
          }
          frame "End" {
            # "Reached when the last step of a macro finishes executing"
            n317 = Unbundle By Name(w719) -> ("n"=w721:i32, "Macro.New.Config.N"=w710:i32)
            n318 = Increment(x=w721) -> (x+1=w718:i32)
            n319 = Greater?(x=w718, y=w710) -> (0:w713:bool)
            n320 = Not Equal?(x=w710, y=-1) -> (x != y?=w712:bool)
            n321 = And(x=w713, y=w712) -> (x .and. y?=w711:bool)
            n322 = Bundle By Name(cluster=w719, "n"=w718) -> (w717:T5)
            n323 = Select(t="Macro: Process >> Complete", s=w711, f="Macro: Process >> Repeat") -> (s? t:f=w715:string)
          }
          frame "Repeat" {
            w722 = 0 ("Step")
            # "Reached when a whole macro needs to be repeated"
            n324 = Bundle By Name(cluster=w725, "Step"=w722, "Rcount"=w722) -> (w724:T5)
          }
          frame "Complete" {
            # "Reached when a macro fully finishes including all repeats"
            n325 = Unbundle By Name(w727) -> ("Macro.New.Config.Activation Type"=w726:enum32{"Hotkey", "Automatic"})
            n326 = case shown="\"Hotkey\"" w726 {
              tunnel: ["Data: Build Report\nUI: Update Status >> Complete Listen\nUI: Listen" "UI: Update Status >> Complete Idle"] -> w728
              frame "Hotkey" {
              }
              frame "Automatic" {
                n327 = property on="Start/Stop" class="Bool (strict)"("Val(Sgnl)"=FALSE ("Value (Signaling)")) -> ()  [unwired: 2 in, 2 out]
              }
            }
          }
          frame "Abort" {
            # "Reached when Abort hotkey is detected"
            n328 = Unbundle By Name(w733) -> ("Macro.New.Config.Activation Type"=w732:enum32{"Hotkey", "Automatic"})
            n329 = case shown="\"Automatic\"" w732 {
              tunnel: ["UI: Update Status >> Abort Listen\nUI: Listen" "UI: Update Status >> Abort Idle"] -> w734
              frame "Hotkey" {
              }
              frame "Automatic" {
                n330 = property on="Start/Stop" class="Bool (strict)"("Val(Sgnl)"=FALSE ("Value (Signaling)")) -> ()  [unwired: 2 in, 2 out]
              }
            }
          }
        }
        n331 = call "Enqueue Multiple States.vi"("queue in"=w669, "State(s) at Back"=w671) -> ()  [unwired: 13 in, 1 out]
      }
      frame "Macro: Exit" {
        # "Exit Macro\n(This is called once, when the VI exits)"
        n332 = Unbundle By Name(w746) -> ("Core.Close Panel on Exit?"=w745:bool)
        n333 = property on="Macro Steps" class="MCListbox (strict)"("TopLeft"=T15 {"Row"=0, "Column"=0} ("Index Values")) -> ()  [unwired: 2 in, 2 out]
        n334 = property on="Macro Steps" class="MCListbox (strict)"("ItemNames"=string[][] [] ("Item Names")) -> ()  [unwired: 2 in, 2 out]
        n335 = Select(t="UI: Front Panel State >> Close", s=w745, f="") -> (s? t:f=w740:string)
        n336 = call "Enqueue Multiple States.vi"("State(s) at Front"=w740, "queue in"=w741, "State(s) at Back"="Data: Cleanup\nExit") -> ()  [unwired: 12 in, 1 out]
      }
      frame "---------- Process ----------" {
      }
      frame "Process: Perform Step" {
        n337 = Unbundle By Name(w755) -> ("Macro.New.Steps"=w763:T8[], "Step"=w751:i32, "Hotkey Values"=w758:T11, "Keyboard"=w759:refnum<k1>)
        n338 = Index Array(array=w763, index=w751) -> (element=w757:T8)
        n339 = call "Perform Step.vi"("error in (no error)"=w761, "Keyboard"=w759, "Hotkeys"=w758, "Step"=w757) -> ("error out"=w760:errorcluster, "Report Data"=w753:T13, "State(s)"=w756:string)  [unwired: 5 in]
        n340 = Number To Decimal String(number=w751) -> (decimal integer string=w752:string)  [unwired: 1 in]
        n341 = Bundle By Name(cluster=w753, "Step"=w752) -> (w750:T13)
        n342 = in-place {
          in-place-border: w750 -> [w764]
          n343 = in-place-cluster #5(w755) -> ("Report Data"=w766:T13[])
          n344 = Build Array (concatenate)(w766, w764) -> (w765:T13[])
          n345 = in-place-cluster #5("Report Data"=w765) -> (w754:T5)
        }
        n346 = call "Enqueue Multiple States.vi"("queue in"=w762, "State(s) at Back"=w756) -> ()  [unwired: 13 in, 1 out]
      }
    }
  }
  n347 = Merge Errors(w9, w8) -> (w10:errorcluster)
  n348 = Release Queue(queue=w11, error in (no error)=w10) -> (error out=→"error out":errorcluster)  [unwired: 1 in, 2 out]
